vi "Get_Auth_Code.vi"(8 "error in (no error)":errorcluster, 11 "OAuth in":refnum<class "OAuth.lvclass">) -> (0 "error out":errorcluster, 3 "OAuth out":refnum<class "OAuth.lvclass">)   [LabVIEW 2016, in "OAuth.lvclass"]
uses:
  OAuth.lvclass
  OAuth.lvclass/OAuth.ctl
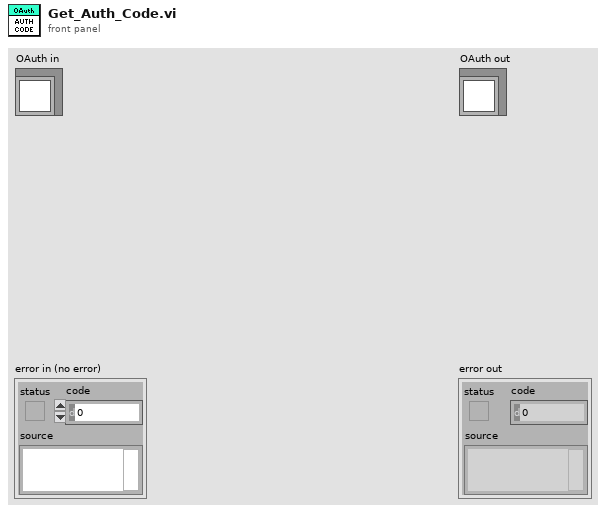
[diagram p1: front panel]
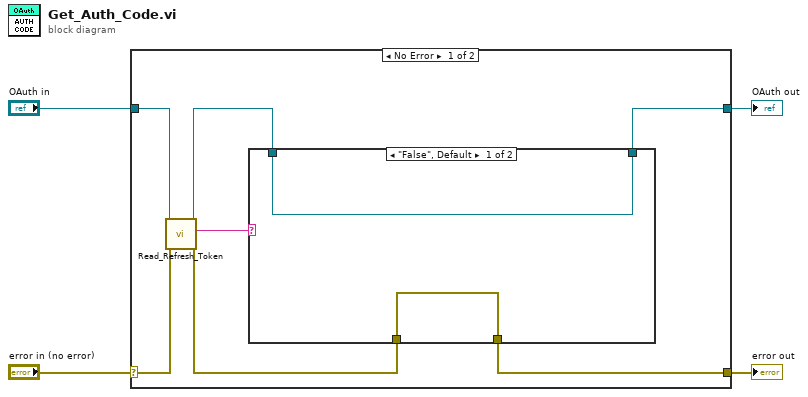
[diagram p0: block diagram]
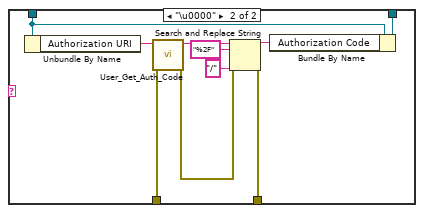
[diagram p2: hidden frame]
diagram:
  n1 = case shown="No Error" "error in (no error)" {
    selector: "error in (no error)" -> [w6 w25]
    tunnel: [w9 w25] -> w3
    tunnel: [w11 w24] -> w1
    tunnel: "OAuth in" -> [w8 w24]
    frame No Error {
      n2 = call-dynamic "Read_Refresh_Token.vi"("error in (no error)"=w6, "OAuth in"=w8) -> ("error out"=w5:errorcluster, "String"=w10:string, "OAuth out"=w7:refnum<class "OAuth.lvclass">)  [unwired: 7 in]
      n3 = case shown="\"False\", Default" w10 {
        tunnel: w5 -> [w13 w19]
        tunnel: w7 -> [w12 w15]
        tunnel: [w12 w14] -> w11
        tunnel: [w13 w18] -> w9
        frame "False", Default {
        }
        frame "\u0000" {
          n4 = Unbundle By Name(w15) -> ("Authorization URI"=w23:string)
          n5 = call "User_Get_Auth_Code.vi"("error in (no error)"=w19, "URL In"=w23) -> ("error out"=w17:errorcluster, "Auth Code"=w20:string)  [unwired: 8 in]
          n6 = Search and Replace String(input string=w20, search string="%2F", replace string="/" ("replace string (\"\")"), error in=w17) -> (result string=w16:string, error out=w18:errorcluster)  [unwired: 4 in, 2 out]
          n7 = Bundle By Name(cluster=w15, "Authorization Code"=w16) -> (w14:refnum<class "OAuth.lvclass">)
        }
      }
    }
    frame Error {
    }
  }
  "error out" <- w3
  "OAuth out" <- w1
